vi "VI_SetWindowPos.vi"(7 "Position(左下)":enum16{"左下", "左上", "居中", "右下", "右上", "正下", "正上"}(ring), 8 "error in (no error)":errorcluster caption="错误输入（无错误）", 10 "Point(CurPos)":cluster{"X":u32, "Y":u32}, 11 "VI REF(本VI)":refnum<vi>) -> (0 "error out":errorcluster caption="错误输出", 3 "VI REF out":refnum<vi>)   [LabVIEW 2016]
uses:
  user32.dll
  <vilib>/Utility/miscctls.llb/LVRectTypeDef.ctl
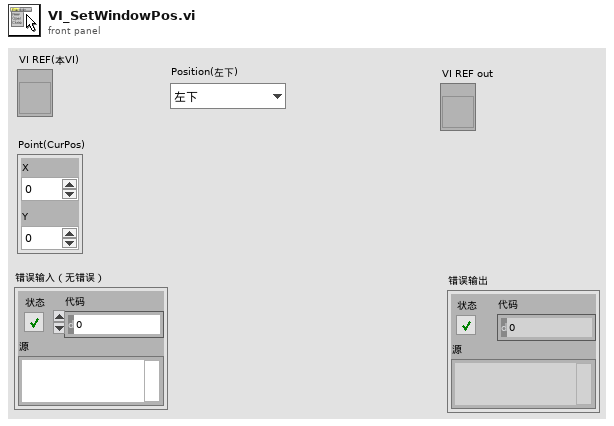
[diagram p1: front panel]
types:
  T1 = enum32{"Invalid", "Standard", "Closed", "Hidden", "Minimized", "Maximized"}
  T2 = typedef "LVRectTypeDef.ctl" = cluster{"Left":i16, "Top":i16, "Right":i16, "Bottom":i16}
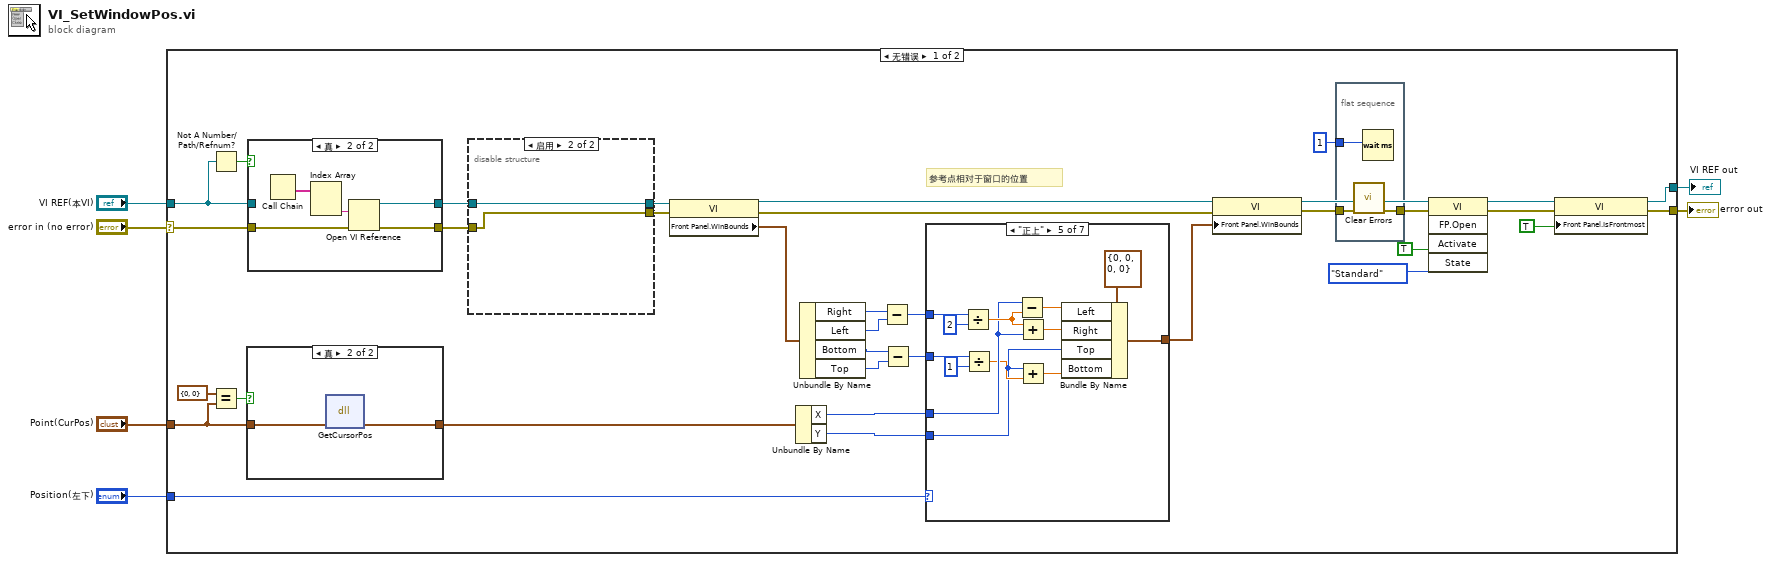
[diagram p0: block diagram]
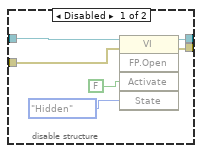
[diagram p2: hidden frame]
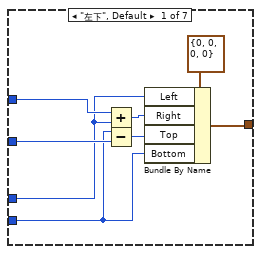
[diagram p3: hidden frame]
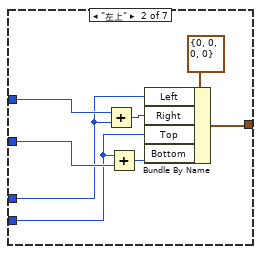
[diagram p4: hidden frame]
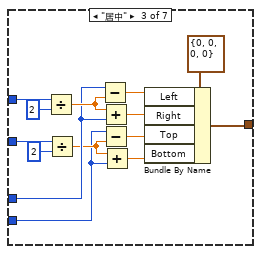
[diagram p5: hidden frame]
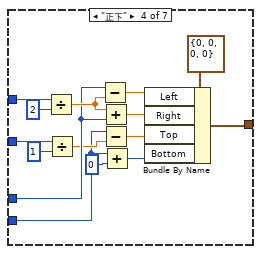
[diagram p6: hidden frame]
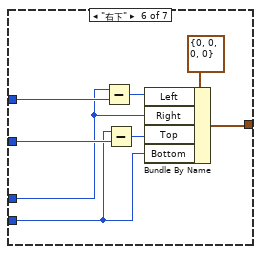
[diagram p7: hidden frame]
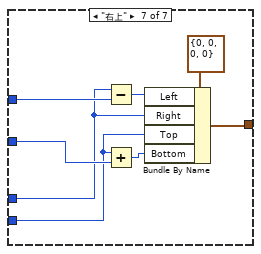
[diagram p8: hidden frame]
diagram:
  n1 = case shown="无错误" "error in (no error)" {
    selector: "error in (no error)" -> [w26 w138]
    tunnel: "VI REF(本VI)" -> [w27 w137]
    tunnel: [w10 w138] -> w5
    tunnel: "Point(CurPos)" -> [w24 _]
    tunnel: "Position(左下)" -> [w22 _]
    tunnel: [w7 w137] -> w1
    frame No Error {
      # "参考点相对于窗口的位置"
      n2 = Not A Number/Path/Refnum?(number/path/refnum=w27) -> (NaN/Path/Refnum?=w28:bool)
      n3 = Equal?(x=cluster{"X":u32, "Y":u32} {"X"=0, "Y"=0}, y=w24) -> (x = y?=w25:bool)
      n4 = case shown="真" w25 {
        tunnel: [w127 w129] -> w41
        tunnel: w24 -> [w127 w128]
        frame False {
        }
        frame True {
          n5 = dll-call lib="user32.dll" fn="GetCursorPos" label="GetCurPos"("lpPoint"=w128) -> ("lpPoint"=w129:cluster{"X":u32, "Y":u32})  [unwired: 3 in, 3 out]
        }
      }
      n6 = case shown="真" w28 {
        tunnel: [w131 w136] -> w18
        tunnel: w27 -> [w131 _]
        tunnel: w26 -> [w130 w133]
        tunnel: [w130 w132] -> w16
        frame False {
        }
        frame True {
          n7 = Call Chain() -> (call chain=w135:string[])
          n8 = Index Array(array=w135) -> (element #2=w134:string)  [unwired: 2 in, 1 out]
          n9 = Open VI Reference(vi path=w134, error in (no error)=w133) -> (vi reference=w136:refnum<vi>, error out=w132:errorcluster)  [unwired: 4 in]
        }
      }
      n10 = disable-structure shown="启用" {
        disable-tunnel: w18 -> [w46 w49]
        disable-tunnel: [w45 w49] -> w17
        disable-tunnel: w16 -> [w44 w48]
        disable-tunnel: [w43 w48] -> w15
        frame Disabled {
          n11 = invoke class="VI" method="FP.Open"(reference=w46, error in=w44, "Activate"=FALSE ("激活？"), "State"=T1."Hidden" ("状态")) -> (reference out=w45:refnum<vi>, error out=w43:errorcluster)  [unwired: 1 in, 3 out]
        }
        frame Enabled {
        }
      }
      n12 = property class="VI"(reference=w17, error in=w15) -> (reference out=w37:refnum<vi>, error out=w38:errorcluster, "Front Panel.WinBounds"=w40:T2)
      n13 = Unbundle By Name(w41) -> ("X"=w30:u32, "Y"=w29:u32)
      n14 = Unbundle By Name(w40) -> ("Right"=w36:i16, "Left"=w35:i16, "Bottom"=w34:i16, "Top"=w33:i16)
      n15 = Subtract(x=w36, y=w35) -> (x-y=w32:i16)
      n16 = Subtract(x=w34, y=w33) -> (x-y=w31:i16)
      n17 = case shown="\"正上\"" w22 {
        tunnel: [w60 w68 w82 w97 w110 w118 w126] -> w39
        tunnel: w32 -> [w59 w67 w80 w95 w108 w117 w125]
        tunnel: w31 -> [w57 w65 w77 w92 w105 w116 w124]
        tunnel: w30 -> [w56 w64 w75 w90 w103 w112 w119]
        tunnel: w29 -> [w54 w62 w70 w84 w99 w114 w121]
        frame "左下", Default {
          n18 = Add(x=w59, y=w56) -> (x+y=w58:u32)
          n19 = Subtract(x=w54, y=w57) -> (x-y=w55:u32)
          n20 = Bundle By Name(cluster=T2 {"Left"=0, "Top"=0, "Right"=0, "Bottom"=0} ("前面板窗口:窗口边界"), "Left"=w56, "Right"=w58, "Top"=w55, "Bottom"=w54) -> (w60:T2)
        }
        frame "左上" {
          n21 = Add(x=w67, y=w64) -> (x+y=w66:u32)
          n22 = Add(x=w62, y=w65) -> (x+y=w61:u32)
          n23 = Bundle By Name(cluster=T2 {"Left"=0, "Top"=0, "Right"=0, "Bottom"=0} ("前面板窗口:窗口边界"), "Left"=w64, "Right"=w66, "Top"=w62, "Bottom"=w61) -> (w68:T2)
        }
        frame "居中" {
          n24 = Divide(x=w80, y=i16 2) -> (x/y=w76:dbl)
          n25 = Divide(x=w77, y=i16 2) -> (x/y=w71:dbl)
          n26 = Subtract(x=w75, y=w76) -> (x-y=w73:dbl)
          n27 = Add(x=w76, y=w75) -> (x+y=w74:dbl)
          n28 = Subtract(x=w70, y=w71) -> (x-y=w69:dbl)
          n29 = Add(x=w71, y=w70) -> (x+y=w72:dbl)
          n30 = Bundle By Name(cluster=T2 {"Left"=0, "Top"=0, "Right"=0, "Bottom"=0} ("前面板窗口:窗口边界"), "Left"=w73, "Right"=w74, "Top"=w69, "Bottom"=w72) -> (w82:T2)
        }
        frame "正下" {
          n31 = Divide(x=w95, y=i16 2) -> (x/y=w91:dbl)
          n32 = Divide(x=w92, y=i16 1) -> (x/y=w86:dbl)
          n33 = Subtract(x=w90, y=w91) -> (x-y=w88:dbl)
          n34 = Add(x=w91, y=w90) -> (x+y=w89:dbl)
          n35 = Subtract(x=w84, y=w86) -> (x-y=w85:dbl)
          n36 = Add(x=w84, y=u32 0) -> (x+y=w87:u32)
          n37 = Bundle By Name(cluster=T2 {"Left"=0, "Top"=0, "Right"=0, "Bottom"=0} ("前面板窗口:窗口边界"), "Left"=w88, "Right"=w89, "Top"=w85, "Bottom"=w87) -> (w97:T2)
        }
        frame "正上" {
          n38 = Divide(x=w108, y=i16 2) -> (x/y=w104:dbl)
          n39 = Divide(x=w105, y=i16 1) -> (x/y=w100:dbl)
          n40 = Subtract(x=w103, y=w104) -> (x-y=w101:dbl)
          n41 = Add(x=w104, y=w103) -> (x+y=w102:dbl)
          n42 = Add(x=w99, y=w100) -> (x+y=w98:dbl)
          n43 = Bundle By Name(cluster=T2 {"Left"=0, "Top"=0, "Right"=0, "Bottom"=0} ("前面板窗口:窗口边界"), "Left"=w101, "Right"=w102, "Top"=w99, "Bottom"=w98) -> (w110:T2)
        }
        frame "右下" {
          n44 = Subtract(x=w112, y=w117) -> (x-y=w111:u32)
          n45 = Subtract(x=w114, y=w116) -> (x-y=w115:u32)
          n46 = Bundle By Name(cluster=T2 {"Left"=0, "Top"=0, "Right"=0, "Bottom"=0} ("前面板窗口:窗口边界"), "Left"=w111, "Right"=w112, "Top"=w115, "Bottom"=w114) -> (w118:T2)
        }
        frame "右上" {
          n47 = Subtract(x=w119, y=w125) -> (x-y=w122:u32)
          n48 = Add(x=w121, y=w124) -> (x+y=w120:u32)
          n49 = Bundle By Name(cluster=T2 {"Left"=0, "Top"=0, "Right"=0, "Bottom"=0} ("前面板窗口:窗口边界"), "Left"=w122, "Right"=w119, "Top"=w121, "Bottom"=w120) -> (w126:T2)
        }
      }
      n50 = property class="VI"(reference=w37, error in=w38, "Front Panel.WinBounds"=w39) -> (reference out=w21:refnum<vi>, error out=w14:errorcluster)
      n51 = flat-sequence {
        tunnel: w14 -> [w51]
        tunnel: [w50] -> w13
        tunnel: 1 -> [w52]
        frame #0 {
          n52 = call <vilib>:"Clear Errors.vi"("error in (no error)"=w51) -> ("error out"=w50:errorcluster)  [unwired: 5 in, 1 out]
          n53 = Wait (ms)(milliseconds to wait=w52) -> ()  [unwired: 1 out]
        }
      }
      n54 = invoke class="VI" method="FP.Open"(reference=w21, error in=w13, "Activate"=TRUE ("激活？"), "State"=T1."Standard" ("状态")) -> (reference out=w8:refnum<vi>, error out=w11:errorcluster)  [unwired: 1 in, 3 out]
      n55 = property class="VI"(reference=w8, error in=w11, "Front Panel.IsFrontmost"=TRUE ("前面板窗口:在最前")) -> (reference out=w7:refnum<vi>, error out=w10:errorcluster)
    }
    frame Error {
    }
  }
  "error out" <- w5
  "VI REF out" <- w1
